vi "SearchPosBeAttacked.vi"(1 "Black/White (T/F)":bool, 2 "Board":i32[][](array[numeric])=[[-3, -5, -4, -1, -2, -4, -5, -3], [-6, -6, -6, -6, -6, -6, -6, -6], [0, 0, 0, 0, 0, 0, 0, 0], [0, 0, 0, 0, 0, 0, 0, 0], [0, 0, 0, 0, 0, 0, 0, 0], [0, 0, 0, 0, 0, 0, 0, 0], [6, 6, 6, 6, 6, 6, 6, 6], [3, 5, 4, 1, 2, 4, 5, 3]]) -> (0 "AttackablePosition":bool[][](array[boolean]))   [LabVIEW 2014]
doc: "Search all positions can be attacked by tthe team.\nInput true: search pos can be attacked by black\nInput false: search pos can be attacked by white"
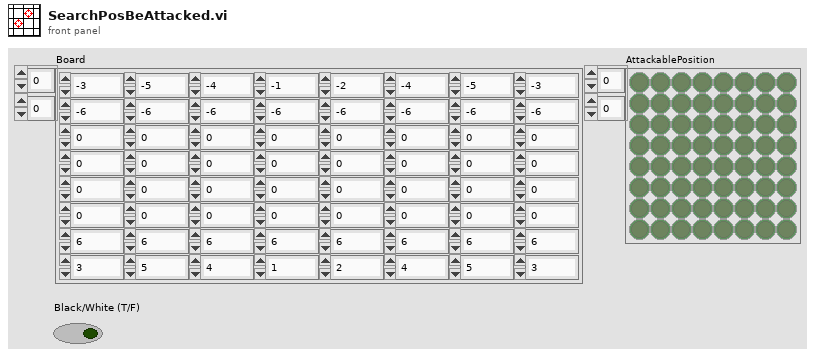
[diagram p1: front panel]
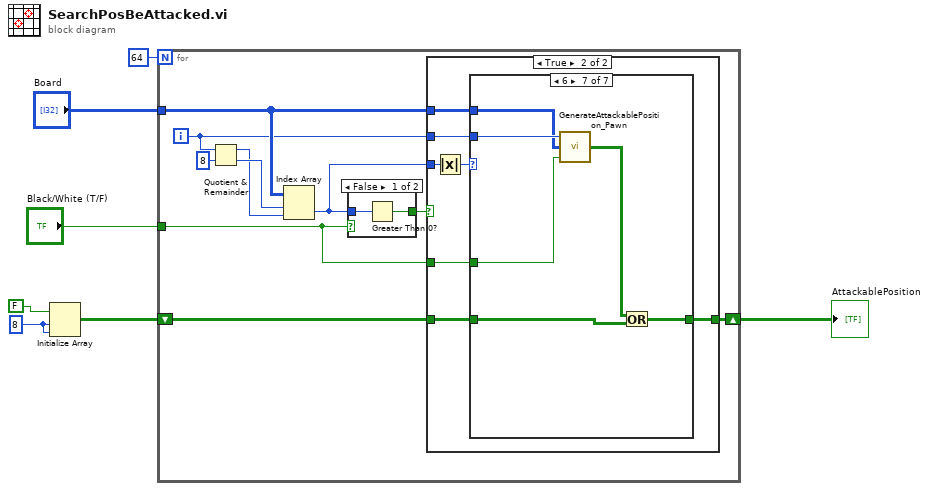
[diagram p0: block diagram]
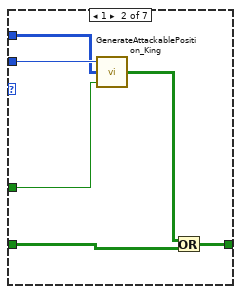
[diagram p4: hidden frame]
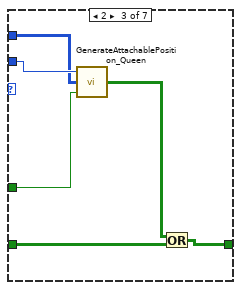
[diagram p5: hidden frame]
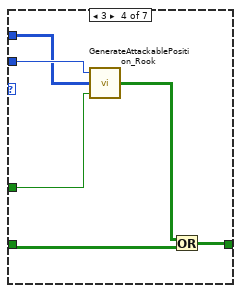
[diagram p6: hidden frame]
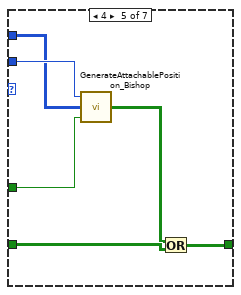
[diagram p7: hidden frame]
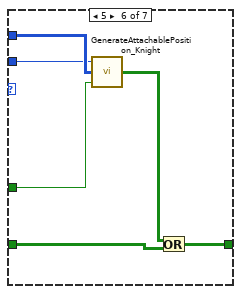
[diagram p8: hidden frame]
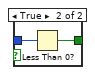
[diagram p9: hidden frame]
diagram:
  w4 = 8 ("dimension size")
  n1 = Initialize Array(FALSE, w4, w4) -> (w2:bool[][])
  n2 = for {
    N: 64 -> [_]
    tunnel: "Board" -> [w15]
    tunnel: "Black/White (T/F)" -> [w9]
    shift-right: [w13] -> w1
    shift-left: w2 -> [w14]
    i -> [w8]
    n3 = Quotient & Remainder(x=w8, y=8) -> (x-y*floor(x/y)=w10:i32, floor(x/y)=w11:i32)
    n4 = Index Array(array=w15, index (row)=w11, index (col)=w10) -> (element=w12:i32)
    n5 = case shown="False" w9 {
      tunnel: w12 -> [w64 w66]
      tunnel: [w63 w65] -> w16
      frame False {
        n6 = Greater Than 0?(x=w64) -> (x > 0?=w63:bool)
      }
      frame True {
        n7 = Less Than 0?(x=w66) -> (x < 0?=w65:bool)
      }
    }
    n8 = case shown="True" w16 {
      tunnel: w15 -> [_ w23]
      tunnel: w14 -> [w18 w22]
      tunnel: [w18 w21] -> w13
      tunnel: w12 -> [_ w25]
      tunnel: w9 -> [_ w20]
      tunnel: w8 -> [_ w19]
      frame False {
      }
      frame True {
        n9 = Absolute Value(x=w25) -> (abs(x)=w24:i32)
        n10 = case shown="6" w24 {
          tunnel: w23 -> [_ w31 w36 w43 w49 w55 w59]
          tunnel: w22 -> [w26 w27 w35 w40 w46 w56 w61]
          tunnel: [w26 w29 w33 w41 w47 w52 w62] -> w21
          tunnel: w20 -> [_ w30 w38 w42 w48 w53 w58]
          tunnel: w19 -> [_ w32 w37 w44 w50 w54 w60]
          frame 0, Default {
          }
          frame 1 {
            n11 = call "GenerateAttackablePosition_King.vi"("Black/White Turn (T/F)"=w30, "Board"=w31, "pieceIndex"=w32) -> ("AttackablePosition"=w28:bool[][])
            n12 = Or(x=w28, y=w27) -> (x .or. y?=w29:bool[][])
          }
          frame 2 {
            n13 = call "GenerateAttachablePosition_Queen.vi"("Black/White Turn (T/F)"=w38, "Board"=w36, "pieceIndex"=w37) -> ("AttachablePosition"=w34:bool[][])
            n14 = Or(x=w34, y=w35) -> (x .or. y?=w33:bool[][])
          }
          frame 3 {
            n15 = call "GenerateAttackablePosition_Rook.vi"("Black/White Turn (T/F)"=w42, "Board"=w43, "pieceIndex"=w44) -> ("AttachablePosition"=w39:bool[][])
            n16 = Or(x=w39, y=w40) -> (x .or. y?=w41:bool[][])
          }
          frame 4 {
            n17 = call "GenerateAttachablePosition_Bishop.vi"("Black/White Turn (T/F)"=w48, "Board"=w49, "pieceIndex"=w50) -> ("AttachablePosition"=w45:bool[][])
            n18 = Or(x=w45, y=w46) -> (x .or. y?=w47:bool[][])
          }
          frame 5 {
            n19 = call "GenerateAttachablePosition_Knight.vi"("Black/White Turn (T/F)"=w53, "Board"=w55, "pieceIndex"=w54) -> ("AttachablePosition"=w51:bool[][])
            n20 = Or(x=w51, y=w56) -> (x .or. y?=w52:bool[][])
          }
          frame 6 {
            n21 = call "GenerateAttackablePosition_Pawn.vi"("Black/White (T/F)"=w58, "Board"=w59, "pieceIndex"=w60) -> ("AttackablePosition"=w57:bool[][])
            n22 = Or(x=w57, y=w61) -> (x .or. y?=w62:bool[][])
          }
        }
      }
    }
  }
  "AttackablePosition" <- w1
